vi "Clear Index.vi"(8 "error in (no error)":errorcluster, 11 "Indexing Test Finder in":refnum<class "Indexing Test Finder.lvclass">) -> (0 "error out":errorcluster, 3 "Indexing Test Finder out":refnum<class "Indexing Test Finder.lvclass">)   [LabVIEW 2020, in "Indexing Test Finder.lvclass"]
uses:
  Indexing Test Finder.lvclass
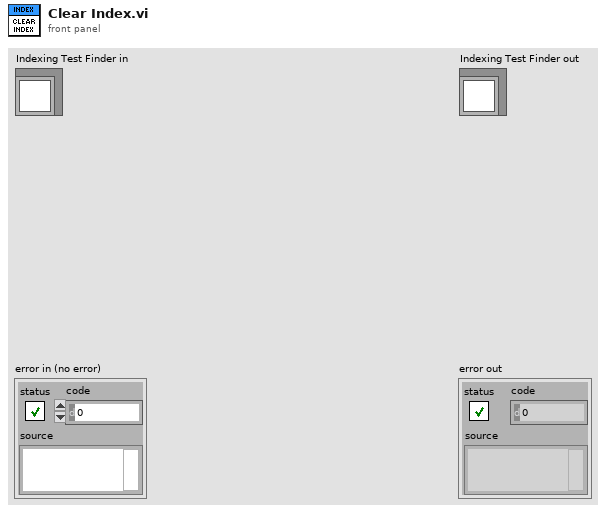
[diagram p1: front panel]
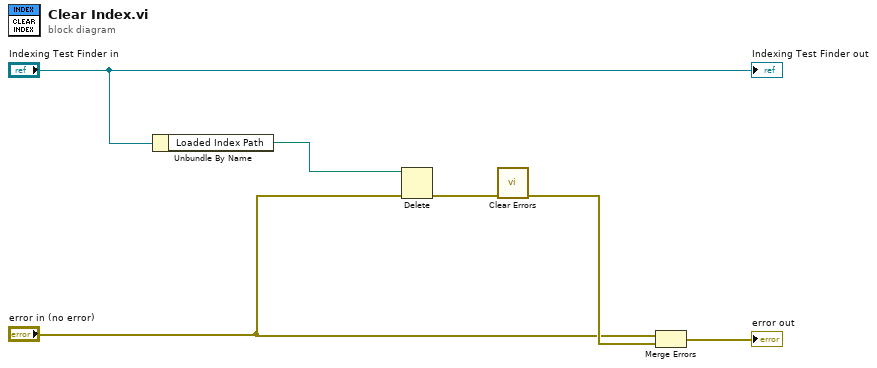
[diagram p0: block diagram]
diagram:
  n1 = Unbundle By Name("Indexing Test Finder in") -> ("Loaded Index Path"=w1:path)
  n2 = Delete(path (use dialog)=w1, error in="error in (no error)") -> (error out=w6:errorcluster)  [unwired: 3 in, 2 out]
  n3 = call <vilib>:"Clear Errors.vi"("error in (no error)"=w6) -> ("error out"=w5:errorcluster)  [unwired: 5 in, 1 out]
  n4 = Merge Errors("error in (no error)", w5) -> (→"error out":errorcluster)
  "Indexing Test Finder out" <- "Indexing Test Finder in"
